vi "HDF5_Write_TE_Record.vi"(0 "HealthRefs":T2 {"TimeStamp" format="%.0x"; "TE_Outp3_dset" format="%.0x"; "TE_Temp3_dset" format="%.0x"; "TE_Outp2_dset" format="%.0x"; "TE_Temp2_dset" format="%.0x"; "TE_Outp1_dset" format="%.0x"; "TE_Temp1_dset" format="%.0x"; "Group_ref" format="%.0x"}, 7 "Health_TE":T1, 11 "error in":errorcluster) -> (15 "error out":errorcluster)   [LabVIEW 2018]
doc: "Write a single Noise<x> record with timestamp:\nNoise1\n NoiseInfo - cluster with Timestamp and other metadata for this record\n SummdSpectrum - 1024 element Double array (waveform)"
uses:
  HDF5_Health_Refs.ctl
  <vilib>/addons/h5labview2/base/hid_t.ctl
  Controls/Clusts/TE_Data_Clust.ctl
  <vilib>/addons/h5labview2/base/lib_path.vi
  <vilib>/addons/h5labview2/base/H5Equery.vi
  lib_path_mod_20200519.vi
  <vilib>/addons/h5labview2/dataset/H5Dwrite.llb/H5Dwrite.xnode
  <vilib>/addons/h5labview2/dataset/H5D.lvlib
  <vilib>/addons/h5labview2/space/H5S.lvlib
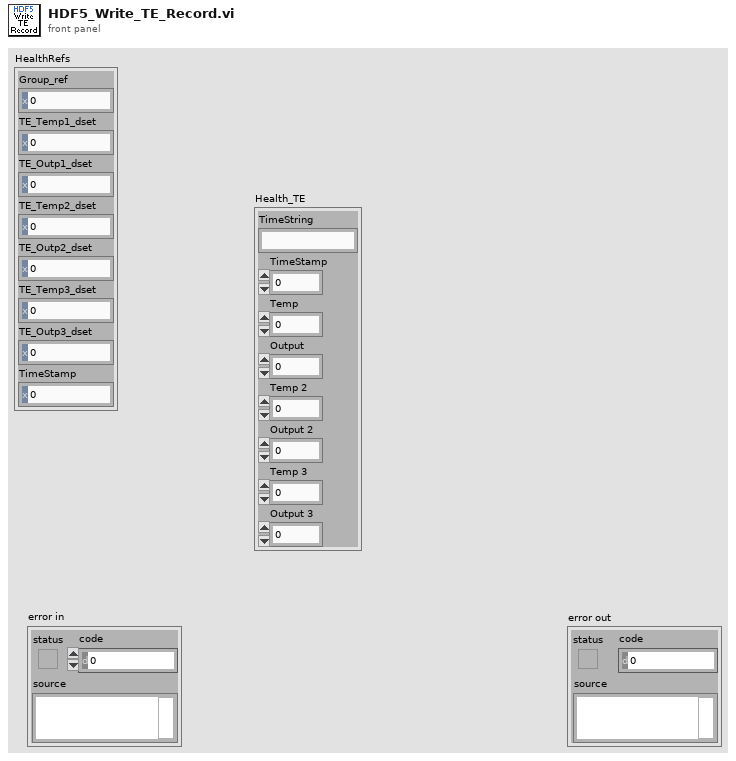
[diagram p1: front panel]
types:
  T1 = typedef "TE_Data_Clust.ctl" = cluster{"TimeString":string, "TimeStamp":dbl, "Temp":dbl, "Output":dbl, "Temp 2":dbl, "Output 2":dbl, "Temp 3":dbl, "Output 3":dbl}
  T2 = typedef "HDF5_Health_Refs.ctl" = cluster{"Group_ref":T3, "TE_Temp1_dset":T3, "TE_Outp1_dset":T3, "TE_Temp2_dset":T3, "TE_Outp2_dset":T3, "TE_Temp3_dset":T3, "TE_Outp3_dset":T3, "TimeStamp":T3}
  T3 = typedef "hid_t.ctl" = i32
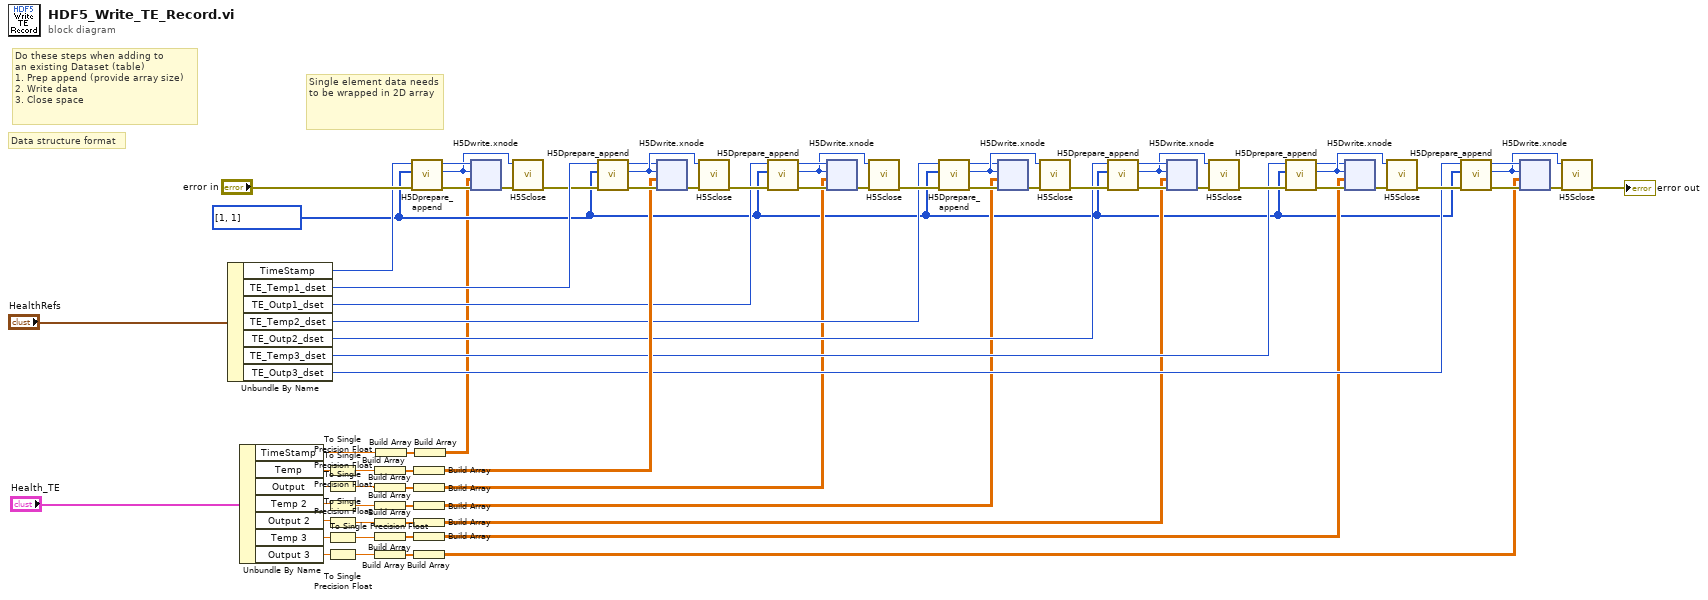
[diagram p0: block diagram]
diagram:
  w5 = u64[] [1, 1] ("append dims")
  # "Single element data needs to be wrapped in 2D array"
  # "Data structure format"
  # "Do these steps when adding to \nan existing Dataset (table)\n1. Prep append (provide array size)\n2. Write data\n3. Close space"
  n1 = Unbundle By Name("HealthRefs") -> ("TimeStamp"=w6:T3, "TE_Temp1_dset"=w24:T3, "TE_Outp1_dset"=w23:T3, "TE_Temp2_dset"=w22:T3, "TE_Outp2_dset"=w21:T3, "TE_Temp3_dset"=w20:T3, "TE_Outp3_dset"=w19:T3)
  n2 = Unbundle By Name("Health_TE") -> ("TimeStamp"=w2:dbl, "Temp"=w66:dbl, "Output"=w55:dbl, "Temp 2"=w56:dbl, "Output 2"=w57:dbl, "Temp 3"=w58:dbl, "Output 3"=w59:dbl)
  n3 = To Single Precision Float(number=w66) -> (single precision float=w65:sgl)
  n4 = To Single Precision Float(number=w55) -> (single precision float=w54:sgl)
  n5 = To Single Precision Float(number=w56) -> (single precision float=w53:sgl)
  n6 = To Single Precision Float(number=w57) -> (single precision float=w52:sgl)
  n7 = To Single Precision Float(number=w58) -> (single precision float=w51:sgl)
  n8 = To Single Precision Float(number=w59) -> (single precision float=w50:sgl)
  n9 = Build Array(w65) -> (w69:sgl[])
  n10 = Build Array(w54) -> (w64:sgl[])
  n11 = Build Array(w53) -> (w63:sgl[])
  n12 = Build Array(w52) -> (w62:sgl[])
  n13 = Build Array(w51) -> (w61:sgl[])
  n14 = Build Array(w50) -> (w60:sgl[])
  n15 = Build Array(w2) -> (w4:dbl[])
  n16 = call <vilib>:"H5Dprepare_append.vi"("error in (no error)"="error in", "append dims"=w5, "dset in"=w6) -> ("error out"=w9:errorcluster, "space out"=w11:T3, "dset out"=w12:T3)  [unwired: 5 in, 1 out]
  n17 = Build Array(w69) -> (w67:sgl[][])
  n18 = Build Array(w64) -> (w17:sgl[][])
  n19 = Build Array(w63) -> (w16:sgl[][])
  n20 = Build Array(w62) -> (w15:sgl[][])
  n21 = Build Array(w61) -> (w14:sgl[][])
  n22 = Build Array(w60) -> (w13:sgl[][])
  n23 = Build Array(w4) -> (w3:dbl[][])
  n24 = xnode "H5Dwrite.xnode"("error in (no error)"=w9, "data"=w3, "file space"=w11, "ref in"=w12) -> ("error out"=w10:errorcluster)  [unwired: 3 in, 2 out]
  n25 = call <vilib>:"H5Sclose.vi"("error in (no error)"=w10, "space in"=w11) -> ("error out"=w8:errorcluster)  [unwired: 9 in]
  n26 = call <vilib>:"H5Dprepare_append.vi"("error in (no error)"=w8, "append dims"=w5, "dset in"=w24) -> ("error out"=w73:errorcluster, "space out"=w71:T3, "dset out"=w70:T3)  [unwired: 5 in, 1 out]
  n27 = xnode "H5Dwrite.xnode"("error in (no error)"=w73, "data"=w67, "file space"=w71, "ref in"=w70) -> ("error out"=w72:errorcluster)  [unwired: 3 in, 2 out]
  n28 = call <vilib>:"H5Sclose.vi"("error in (no error)"=w72, "space in"=w71) -> ("error out"=w33:errorcluster)  [unwired: 9 in]
  n29 = call <vilib>:"H5Dprepare_append.vi"("error in (no error)"=w33, "append dims"=w5, "dset in"=w23) -> ("error out"=w46:errorcluster, "space out"=w48:T3, "dset out"=w49:T3)  [unwired: 5 in, 1 out]
  n30 = xnode "H5Dwrite.xnode"("error in (no error)"=w46, "data"=w17, "file space"=w48, "ref in"=w49) -> ("error out"=w47:errorcluster)  [unwired: 3 in, 2 out]
  n31 = call <vilib>:"H5Sclose.vi"("error in (no error)"=w47, "space in"=w48) -> ("error out"=w32:errorcluster)  [unwired: 9 in]
  n32 = call <vilib>:"H5Dprepare_append.vi"("error in (no error)"=w32, "append dims"=w5, "dset in"=w22) -> ("error out"=w45:errorcluster, "space out"=w43:T3, "dset out"=w42:T3)  [unwired: 5 in, 1 out]
  n33 = xnode "H5Dwrite.xnode"("error in (no error)"=w45, "data"=w16, "file space"=w43, "ref in"=w42) -> ("error out"=w44:errorcluster)  [unwired: 3 in, 2 out]
  n34 = call <vilib>:"H5Sclose.vi"("error in (no error)"=w44, "space in"=w43) -> ("error out"=w31:errorcluster)  [unwired: 9 in]
  n35 = call <vilib>:"H5Dprepare_append.vi"("error in (no error)"=w31, "append dims"=w5, "dset in"=w21) -> ("error out"=w38:errorcluster, "space out"=w40:T3, "dset out"=w41:T3)  [unwired: 5 in, 1 out]
  n36 = xnode "H5Dwrite.xnode"("error in (no error)"=w38, "data"=w15, "file space"=w40, "ref in"=w41) -> ("error out"=w39:errorcluster)  [unwired: 3 in, 2 out]
  n37 = call <vilib>:"H5Sclose.vi"("error in (no error)"=w39, "space in"=w40) -> ("error out"=w30:errorcluster)  [unwired: 9 in]
  n38 = call <vilib>:"H5Dprepare_append.vi"("error in (no error)"=w30, "append dims"=w5, "dset in"=w20) -> ("error out"=w29:errorcluster, "space out"=w37:T3, "dset out"=w36:T3)  [unwired: 5 in, 1 out]
  n39 = xnode "H5Dwrite.xnode"("error in (no error)"=w29, "data"=w14, "file space"=w37, "ref in"=w36) -> ("error out"=w28:errorcluster)  [unwired: 3 in, 2 out]
  n40 = call <vilib>:"H5Sclose.vi"("error in (no error)"=w28, "space in"=w37) -> ("error out"=w27:errorcluster)  [unwired: 9 in]
  n41 = call <vilib>:"H5Dprepare_append.vi"("error in (no error)"=w27, "append dims"=w5, "dset in"=w19) -> ("error out"=w26:errorcluster, "space out"=w34:T3, "dset out"=w35:T3)  [unwired: 5 in, 1 out]
  n42 = xnode "H5Dwrite.xnode"("error in (no error)"=w26, "data"=w13, "file space"=w34, "ref in"=w35) -> ("error out"=w25:errorcluster)  [unwired: 3 in, 2 out]
  n43 = call <vilib>:"H5Sclose.vi"("error in (no error)"=w25, "space in"=w34) -> ("error out"=→"error out":errorcluster)  [unwired: 9 in]
